vi "PlotMePe.vi"(5 "PePlotRef":refnum<vi>, 7 "MePlotRef":refnum<vi>, 8 "ErrorArray":errorcluster[](array[cluster]), 10 "clPmuRptArray":T1 {"Synx" format="%#_4g"}, 11 "clEvtReportArray":T1 {"Synx" format="%#_4g"}) -> (0 "ErrorArray":errorcluster[](array[cluster]))   [LabVIEW 2014, in "Visualization.lvlib" / "VisualizePMU_class.lvclass"]
uses:
  VisualizePMU_class.lvclass
  Modules/EventPlugins/EventPluginBaseClass/TypeDefs/clEvtReportArray.ctl
  Modules/EventPlugins/EventPluginBaseClass/TypeDefs/clEvtReport.ctl
  <userlib>/NIST/NISTErrorLib/NISTErrorLib.lvlib
  Modules/EventPlugins/EventPluginBaseClass/EventPluginBaseClass.lvclass
panel:
  out "PE Plot":cluster{dbl[], "TVE":dbl[]}[](graph)
  out "ME Plot":cluster{dbl[], "TVE":dbl[]}[](graph)
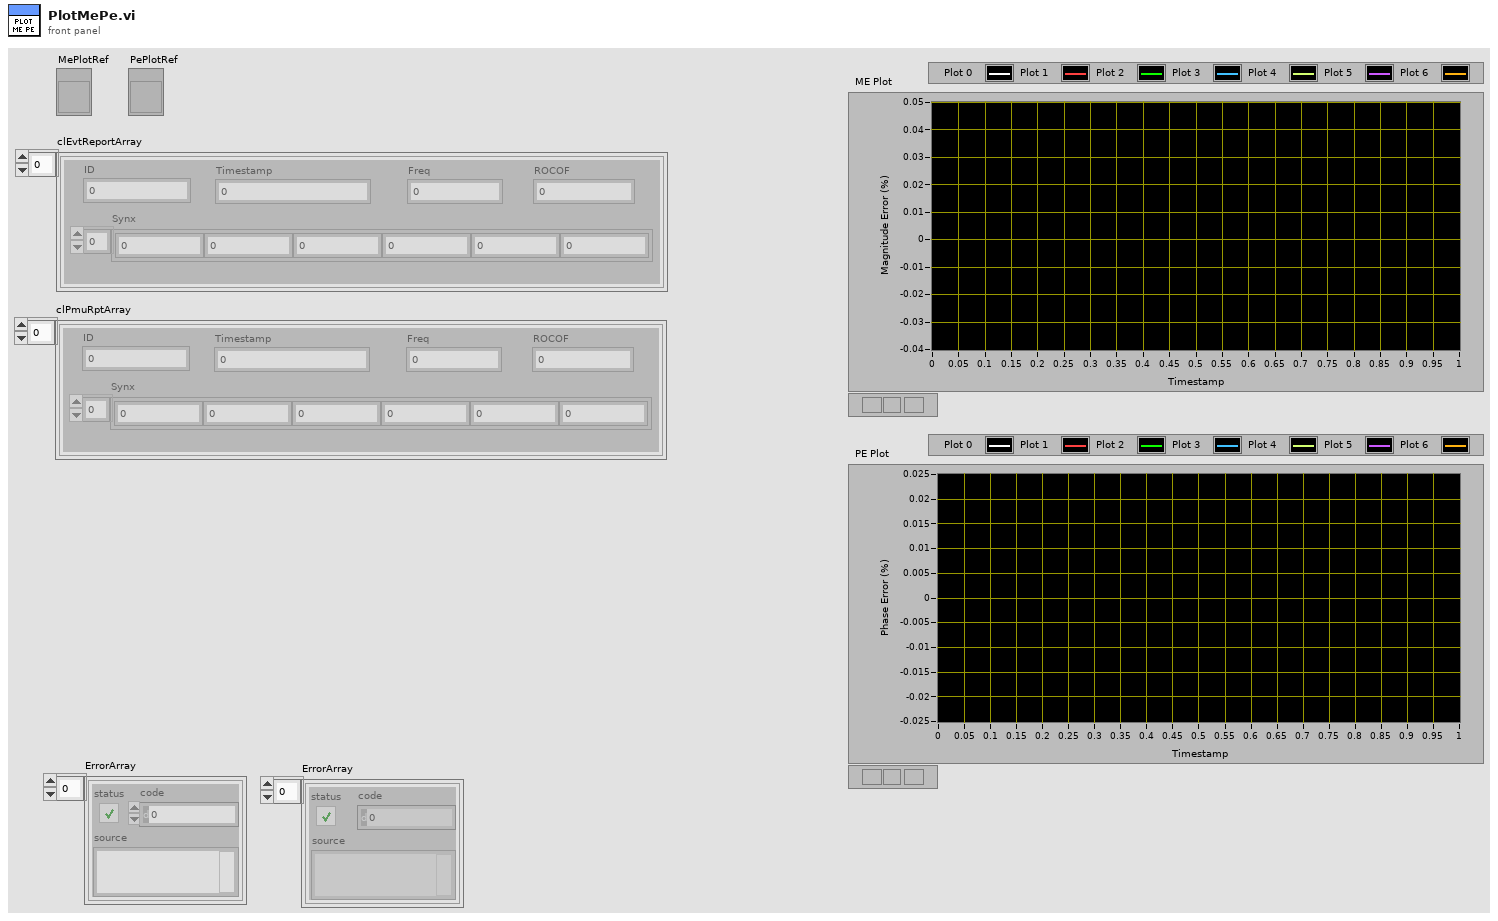
[diagram p1: front panel]
types:
  T1 = typedef "EventPlugins.lvlib/EventPluginBaseClass.lvclass/clEvtReportArray.ctl" = T2[]
  T2 = typedef "EventPlugins.lvlib/EventPluginBaseClass.lvclass/clEvtReport.ctl" = cluster{"Timestamp":dbl, "Synx":cdb[], "Freq":dbl, "ROCOF":dbl, "ID":i16}
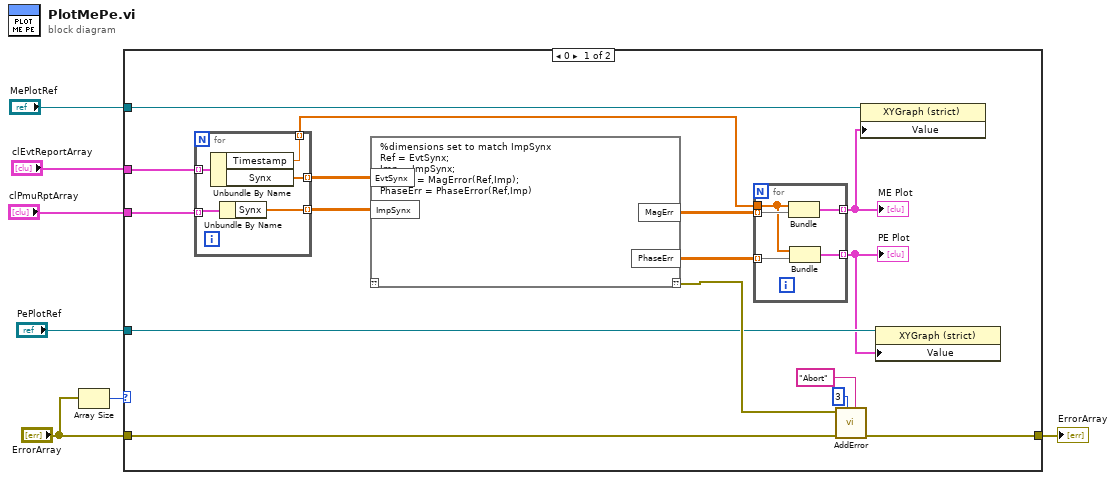
[diagram p0: block diagram]
diagram:
  n1 = Array Size(array="ErrorArray") -> (size(s)=w7:i32)
  n2 = case shown="0" w7 {
    tunnel: "ErrorArray" -> [w13 w34]
    tunnel: [w17 w34] -> w5
    tunnel: "clEvtReportArray" -> [w23 _]
    tunnel: "clPmuRptArray" -> [w22 _]
    tunnel: "MePlotRef" -> [w12 _]
    tunnel: "PePlotRef" -> [w9 _]
    frame 0 {
      n3 = for {
        tunnel: w22 -> [w33] mode=indexing
        tunnel: w23 -> [w32] mode=indexing
        tunnel: [w31] -> w21 mode=indexing
        tunnel: [w30] -> w20 mode=indexing
        tunnel: [w29] -> w18 mode=indexing
        n4 = Unbundle By Name(w32) -> ("Timestamp"=w29:dbl, "Synx"=w31:cdb[])
        n5 = Unbundle By Name(w33) -> ("Synx"=w30:cdb[])
      }
      n6 = script code="%dimensions set to match ImpSynx\nRef = EvtSynx;\nImp = ImpSynx;\nMagErr = MagError(Ref,Imp);\nPhaseErr = PhaseError(Ref,Imp)"("EvtSynx"=w21, "ImpSynx"=w20) -> ("??"=w16:errorcluster, "MagErr"=w19:dbl[][], "PhaseErr"=w10:cdb[][])  [unwired: 1 in]
      n7 = for {
        tunnel: w19 -> [w28] mode=indexing
        tunnel: w18 -> [w26]
        tunnel: [w27] -> w11 mode=indexing
        tunnel: w10 -> [w25] mode=indexing
        tunnel: [w24] -> w8 mode=indexing
        n8 = Bundle(w26, w28) -> (w27:cluster{dbl[], dbl[]})  [unwired: 1 in]
        n9 = Bundle(w26, w25) -> (w24:cluster{dbl[], cdb[]})  [unwired: 1 in]
      }
      "ME Plot" <- w11
      "PE Plot" <- w8
      n10 = call <userlib>:"AddError.vi"("Severity"="Abort" ("String"), "Priority"=u8 3, "ErrorArray"=w13, "error in (no error)"=w16) -> ("ErrorArray"=w17:errorcluster[])  [unwired: 6 in, 1 out]
      n11 = property class="XYGraph (strict)"(reference=w12, "Value"=w11) -> ()  [unwired: 1 in, 2 out]
      n12 = property class="XYGraph (strict)"(reference=w9, "Value"=w8) -> ()  [unwired: 1 in, 2 out]
    }
    frame 1, Default {
    }
  }
  "ErrorArray" <- w5
